vi "DataVIS_FormatIntensityScales.vi"(8 "error in (no error)":errorcluster, 9 "Control References":T3, 10 "Decimate Controls":T4={"X Low"=-0.1, "X High"=0.1, "X Step"=4e-05, "Voffset -2T"=0.0} {"X Step" format="%#_6p"; "X High" format="%#_6p"; "X Low" format="%#_6p"}, 11 "State Wire IN":T1) -> (0 "error out":errorcluster, 2 "Vfast values":dbl[](array[numeric]), 3 "State Wire OUT":T1)   [LabVIEW 2016]
uses:
  DataVIS_StateWire.ctl
  <vilib>/Utility/miscctls.llb/LVPointDoubleTypeDef.ctl
  <vilib>/Utility/miscctls.llb/LVOffsetAndMultiplierTypeDef.ctl
panel:
  out "X scale":cluster{dbl, "X Step":dbl}={-0.09995000000000001, "X Step"=5e-05}
  out "Y scale":cluster{"Real Voltage":dbl, dbl}={"Real Voltage"=-1.0, 0.050000000000000044}
  out "Scan names 2":string[](array[string])=["DSA_Vsg1", "B", "B"]
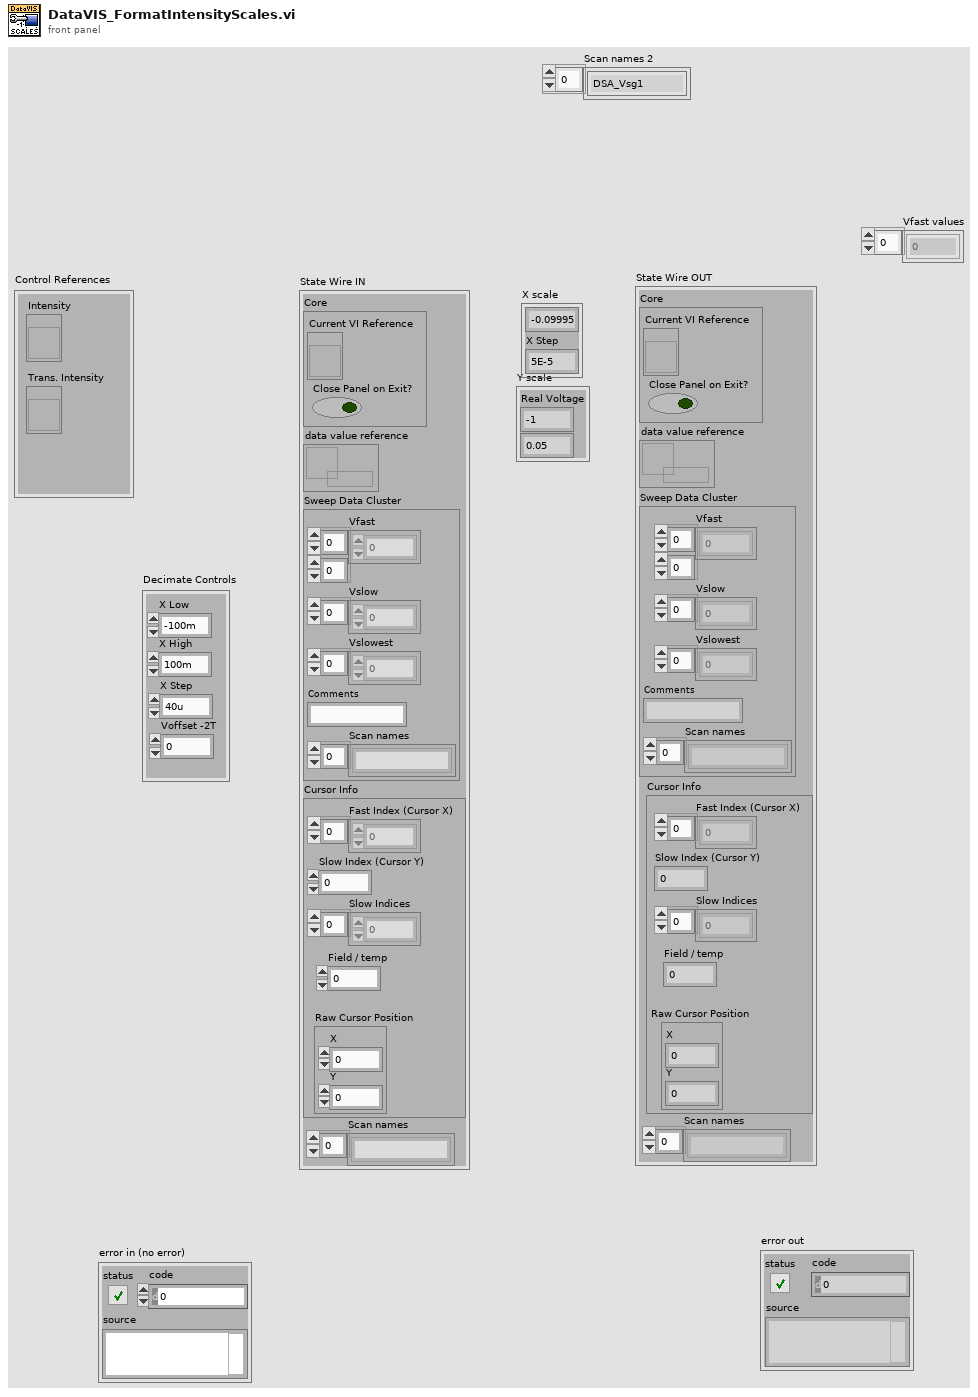
[diagram p1: front panel]
types:
  T1 = typedef "DataVIS_StateWire.ctl" = cluster{"Core":cluster{"Current VI Reference":refnum<vi>, "Close Panel on Exit?":bool}, "data value reference":refnum<data-value>, "Sweep Data Cluster":cluster{"Vfast":dbl[][], "Vslow":dbl[], "Vslowest":dbl[], "Comments":string, "Scan names":string[]}, "Cursor Info":cluster{"Fast Index (Cursor X)":dbl[], "Slow Index (Cursor Y)":dbl, "Slow Indices":dbl[], "Raw Cursor Position":T2, "Field / temp":i32}, "Scan names":string[]}
  T2 = typedef "LVPointDoubleTypeDef.ctl" = cluster{"X":dbl, "Y":dbl}
  T3 = cluster{"Trans. Intensity":refnum<vi>, "Intensity":refnum<vi>}
  T4 = cluster{"X Low":dbl, "X High":dbl, "X Step":dbl, "Voffset -2T":dbl}
  T5 = typedef "LVOffsetAndMultiplierTypeDef.ctl" = cluster{"Offset":dbl, "Multiplier":dbl}
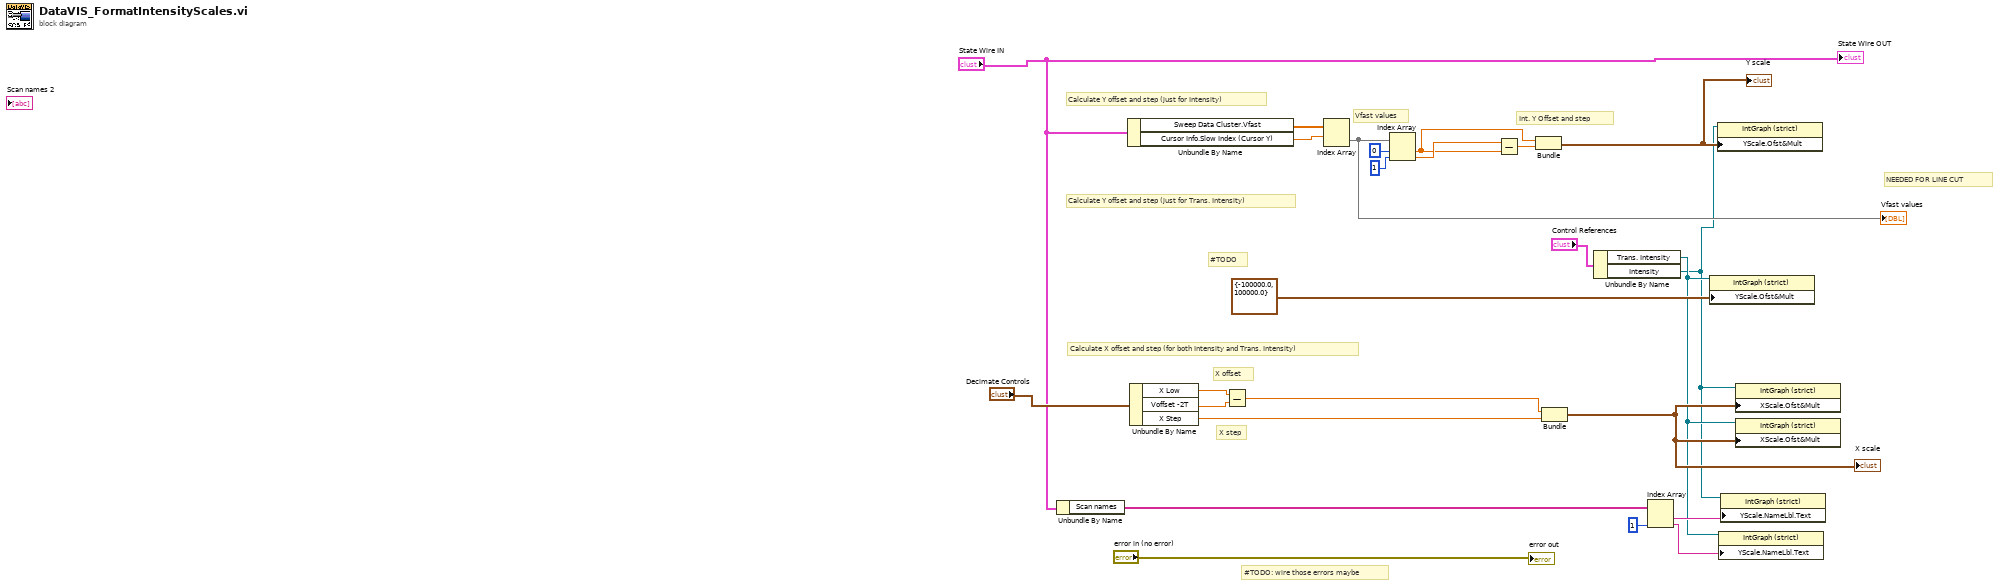
[diagram p0: block diagram]
diagram:
  # "NEEDED FOR LINE CUT"
  # "#TODO: wire those errors maybe"
  # "X step"
  # "X offset"
  # "#TODO"
  # "Calculate Y offset and step (just for Trans. Intensity)"
  # "Calculate X offset and step (for both Intensity and Trans. Intensity)"
  # "Calculate Y offset and step (just for Intensity)"
  # "Int. Y Offset and step"
  # "Vfast values"
  n1 = Unbundle By Name("State Wire IN") -> ("Scan names"=w6:string[])
  n2 = Unbundle By Name("State Wire IN") -> ("Sweep Data Cluster.Vfast"=w15:dbl[][], "Cursor Info.Slow Index (Cursor Y)"=w14:dbl)
  n3 = Unbundle By Name("Decimate Controls") -> ("X Low"=w11:dbl, "Voffset -2T"=w10:dbl, "X Step"=w8:dbl)
  n4 = Subtract(x=w11, y=w10) -> (x-y=w9:dbl)
  n5 = Index Array(array=w15, index (row)=w14) -> (element=w16:dbl[])  [unwired: 1 in]
  "Vfast values" <- w16
  n6 = Index Array(array=w16, index #1=0 ("index"), index #2=1 ("index")) -> (element #1=w18:dbl, element #2=w19:dbl)
  n7 = Subtract(x=w19, y=w18) -> (x-y=w17:dbl)
  n8 = Bundle(w18, w17) -> (w7:cluster{dbl, dbl})  [unwired: 1 in]
  "Y scale" <- w7
  n9 = Bundle(w9, "X Step"=w8) -> (w22:cluster{dbl, "X Step":dbl})  [unwired: 1 in]
  "X scale" <- w22
  n10 = Unbundle By Name("Control References") -> ("Trans. Intensity"=w3:refnum<vi>, "Intensity"=w2:refnum<vi>)
  n11 = Index Array(array=w6, index #2=1 ("index")) -> (element #1=w23:string, element #2=w24:string)  [unwired: 1 in]
  n12 = property on="Property Node" class="IntGraph (strict)"(reference=w3, "YScale.Ofst&Mult"=T5 {"Offset"=-100000.0, "Multiplier"=100000.0} ("Y Scale.Offset and Multiplier")) -> ()  [unwired: 1 in, 2 out]
  n13 = property on="Property Node" class="IntGraph (strict)"(reference=w2, "YScale.Ofst&Mult"=w7) -> ()  [unwired: 1 in, 2 out]
  n14 = property on="Property Node" class="IntGraph (strict)"(reference=w3, "YScale.NameLbl.Text"=w24) -> ()  [unwired: 1 in, 2 out]
  n15 = property on="Property Node" class="IntGraph (strict)"(reference=w2, "YScale.NameLbl.Text"=w23) -> ()  [unwired: 1 in, 2 out]
  n16 = property on="Property Node" class="IntGraph (strict)"(reference=w2, "XScale.Ofst&Mult"=w22) -> ()  [unwired: 1 in, 2 out]
  n17 = property on="Property Node" class="IntGraph (strict)"(reference=w3, "XScale.Ofst&Mult"=w22) -> ()  [unwired: 1 in, 2 out]
  "error out" <- "error in (no error)"
  "State Wire OUT" <- "State Wire IN"
